vi "Read Font Setups.vi"(4 "error in (no error)":errorcluster, 6 "Owner Name":string, 7 "Config Data_DB_ADO in":refnum<class "Config Data_DB_ADO.lvclass">) -> (0 "error out":errorcluster, 1 "Control Names":string[](array[string]), 2 "Font Parameters":cluster{T1[]}[](array[cluster]), 3 "Config Data_DB_ADO out":refnum<class "Config Data_DB_ADO.lvclass">)   [LabVIEW 2020, in "Config Data.lvlib" / "Config Data_DB_ADO.lvclass"]
uses:
  Config Data_DB_ADO.lvclass
  toolbox/ADO Database Drivers/ADO Database Drivers.lvlib
  Config Data_DB.lvclass
  Display Properties Manager/_typedefs/Control Component to Set.ctl
  Display Properties Manager/Display Properties Manager.lvlib
  Display Properties Manager/_typedefs/Font Parameters.ctl
  C:/Users/Fred Guo/Desktop/Release 19/_libraries/Config Data/DB/Config Data_DB.lvclass
  C:/Users/Fred Guo/Desktop/Release 19/_libraries/Config Data/Config Data.lvclass
  C:/Users/Fred Guo/Desktop/Release 19/_libraries/Config Data/DB/ADO/Config Data_DB_ADO.lvclass
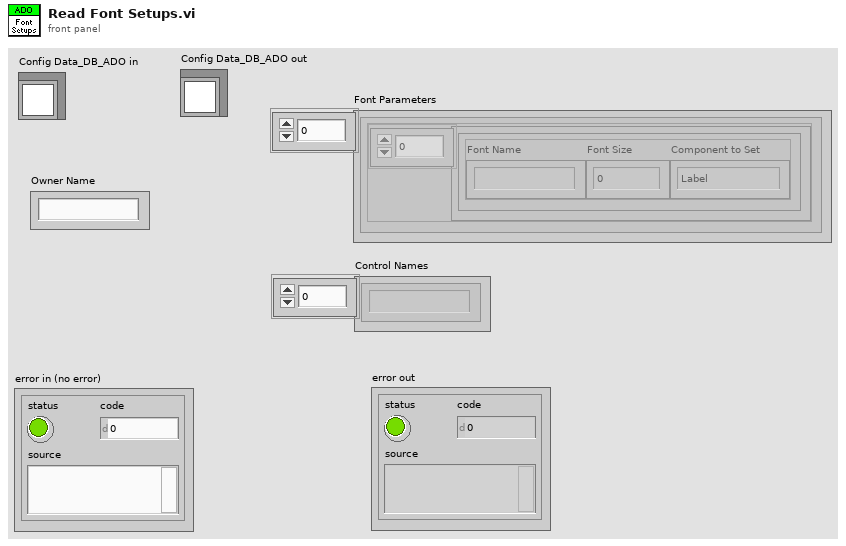
[diagram p1: front panel]
types:
  T1 = typedef "Display Properties Manager.lvlib/Font Parameters.ctl" = cluster{"Font Name":string, "Font Size":u32, "Component to Set":T2}
  T2 = typedef "Display Properties Manager.lvlib/Control Component to Set.ctl" = enum16{"Label", "Caption", "Contents"}
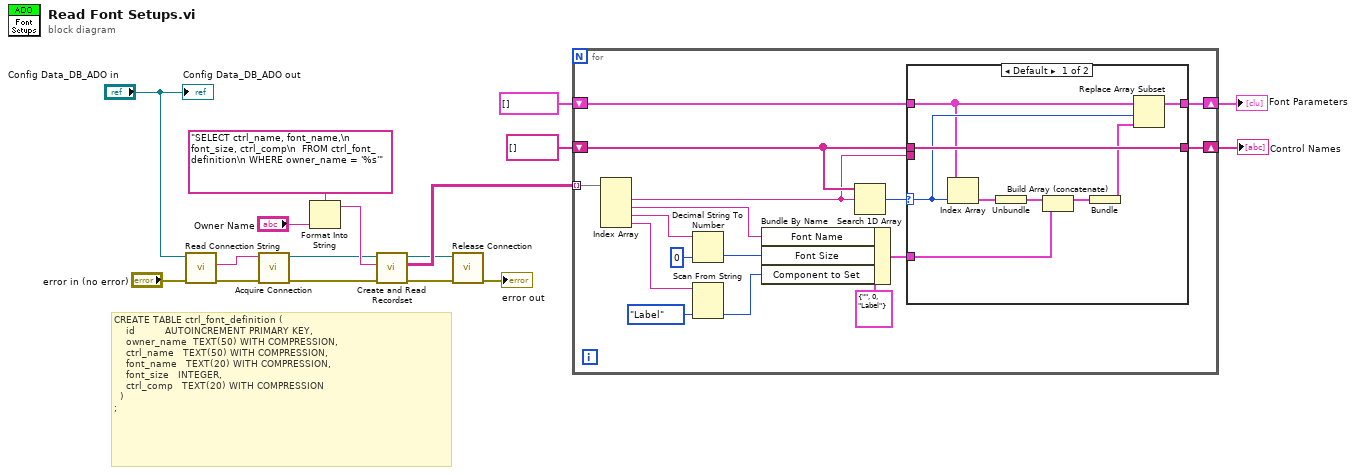
[diagram p0: block diagram]
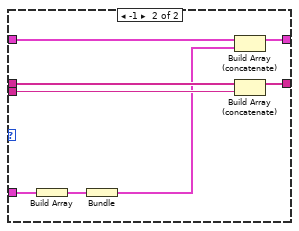
[diagram p2: hidden frame]
diagram:
  # "CREATE TABLE ctrl_font_definition (\n    id          AUTOINCREMENT PRIMARY KEY,\n    owner_name  TEXT(50) WITH COMPRESSION,\n\t   ctrl_name   TEXT(50) WITH COMPRESSION,\n\t   font_name   TEXT(20) WITH COMPRESSION,\n\t   font_size   INTEGER,\n\t   ctrl_comp   TEXT(20) WITH COMPRESSION\n  )\n;"
  n1 = call "Read Connection String.vi"("Error In"="error in (no error)", "DB In"="Config Data_DB_ADO in") -> ("Error Out"=w15:errorcluster, "Connection String"=w16:string)  [unwired: 3 in, 1 out]
  n2 = call "Acquire Connection.vi"("error in (no error)"=w15, "Connection String"=w16) -> ("error out"=w10:errorcluster, "Connection"=w11:refnum<k7>)  [unwired: 3 in, 1 out]
  n3 = Format Into String(format string="SELECT ctrl_name, font_name,\n       font_size, ctrl_comp\n  FROM ctrl_font_definition\n WHERE owner_name = '%s'", "Owner Name") -> (resulting string=w17:string)  [unwired: 2 in, 1 out]
  n4 = call "Create and Read Recordset.vi"("error in (no error)"=w10, "Source"=w17, "Connection In"=w11) -> ("error out"=w2:errorcluster, "DB Data"=w8:string[][], "Connection Out"=w3:refnum<k7>)  [unwired: 2 in, 2 out]
  n5 = call "Release Connection.vi"("error in"=w2, "Connection"=w3) -> ("error out"=→"error out":errorcluster)  [unwired: 5 in]
  n6 = for {
    tunnel: w8 -> [w33] mode=indexing
    shift-right: [w21] -> w6
    shift-left: string[] [] -> [w23]
    shift-right: [w19] -> w4
    shift-left: cluster{T1[]}[] [] -> [w20]
    n7 = Index Array(array=w33) -> (element #1=w22:string, element #2=w31:string, element #3=w30:string, element #4=w27:string)  [unwired: 4 in]
    n8 = Decimal String To Number(string=w30, default (0L)=u32 0 ("default (0 I32)")) -> (number=w29:u32)  [unwired: 1 in, 1 out]
    n9 = Scan From String(input string=w27, default 1=Control_Component_to_Set."Label" ("Component to Set")) -> (output 1=w26:T2)  [unwired: 3 in, 3 out]
    n10 = Bundle By Name(cluster=T1 {"Font Name"="", "Font Size"=0, "Component to Set"=enum."Label"} ("Font Parameters"), "Font Name"=w31, "Font Size"=w29, "Component to Set"=w26) -> (w18:T1)
    n11 = Search 1D Array(1D array=w23, element=w22) -> (index of element=w24:i32)  [unwired: 1 in]
    n12 = case shown="Default" w24 {
      selector: w24 -> [w41 _]
      tunnel: w23 -> [w42 w50]
      tunnel: w22 -> [_ w49]
      tunnel: [w42 w48] -> w21
      tunnel: w20 -> [w40 w47]
      tunnel: [w39 w46] -> w19
      tunnel: w18 -> [w36 w45]
      frame Default {
        n13 = Index Array(array=w40, index=w41) -> (element=w38:cluster{T1[]})
        n14 = Unbundle(w38) -> (w37:T1[])
        n15 = Build Array (concatenate)(w37, w36) -> (w35:T1[])
        n16 = Bundle(w35) -> (w34:cluster{T1[]})  [unwired: 1 in]
        n17 = Replace Array Subset(array=w40, new element=w34, index=w41) -> (w39:cluster{T1[]}[])
      }
      frame -1 {
        n18 = Build Array(w45) -> (w43:T1[])
        n19 = Bundle(w43) -> (w44:cluster{T1[]})  [unwired: 1 in]
        n20 = Build Array (concatenate)(w47, w44) -> (w46:cluster{T1[]}[])
        n21 = Build Array (concatenate)(w50, w49) -> (w48:string[])
      }
    }
  }
  "Font Parameters" <- w4
  "Control Names" <- w6
  "Config Data_DB_ADO out" <- "Config Data_DB_ADO in"
